vi "DetermineTimeSinceLastExecution.vi"(11 "Time Stamp":timestamp) -> (3 "Boolean":bool)   [LabVIEW 2015]
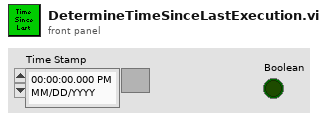
[diagram p1: front panel]
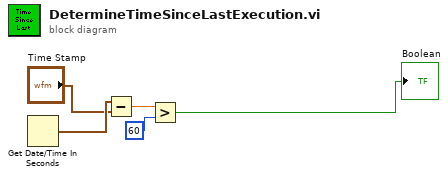
[diagram p0: block diagram]
diagram:
  n1 = Get Date/Time In Seconds() -> (seconds since 1Jan1904=w5:timestamp)
  n2 = Subtract(x=w5, y="Time Stamp") -> (x-y=w3:dbl)
  n3 = Greater?(x=w3, y=60) -> (0:→"Boolean":bool)
